vi "add_int16.vi"   [LabVIEW 2012]
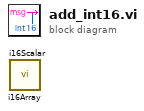
[diagram p0: block diagram]
diagram:
  n1 = call "i16Array.vi"() -> ()  [unwired: 5 in, 1 out]
  n2 = call "i16Scalar.vi"() -> ()  [unwired: 5 in, 1 out]
